vi "New.vi"(1 "Before Write":string) -> (0 "String Writer":refnum<class "String.lvclass">)   [LabVIEW 2018, in "Toolkit.lvlib" / "Writers.lvlib" / "String.lvclass"]
doc: "Creates a new String Writer object.\n\n<B>Before Write</B> - The initial contents of the destination. The rendered Mustache template will be appended to the contents of this value.\n\n<B>String Writer</B> - Represents an implementation capable of writing a rendered Mustache templates to a string."
uses:
  String.lvclass
  String.lvclass/String.ctl
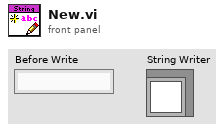
[diagram p1: front panel]
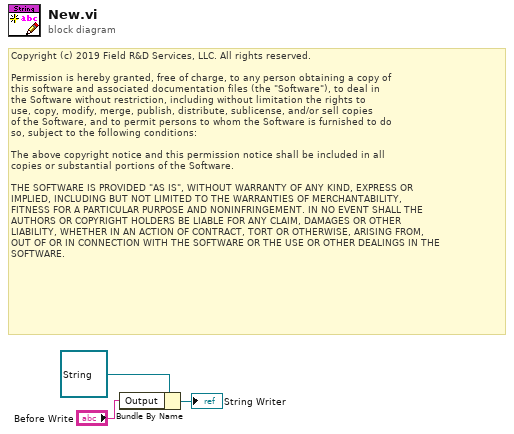
[diagram p0: block diagram]
diagram:
  # "Copyright (c) 2019 Field R&D Services, LLC. All rights reserved.\n\nPermission is hereby granted, free of charge, to any person obtaining a copy of\nthis software and associated documentation files (the \"Software\"), to deal in\nthe Software without restriction, including without limitation the rights to\nuse, copy, modify, merge, publish, distribute, sublicense, and/or sell copies\nof the Software, and to permit persons to whom the Software is furnished to do\nso, subject to the following conditions:\n\nThe above copyright notice and this permission notice shall be included in all\ncopies or substantial portions of the Software.\n\nTHE SOFTWARE IS PROVIDED \"AS IS\", WITHOUT WARRANTY OF ANY KIND, EXPRESS OR\nIMPLIED, INCLUDING BUT NOT LIMITED TO THE WARRANTIES OF MERCHANTABILITY,\nFITNESS FOR A PARTICULAR PURPOSE AND NONINFRINGEMENT. IN NO EVENT SHALL THE\nAUTHORS OR COPYRIGHT HOLDERS BE LIABLE FOR ANY CLAIM, DAMAGES OR OTHER\nLIABILITY, WHETHER IN AN ACTION OF CONTRACT, TORT OR OTHERWISE, ARISING FROM,\nOUT OF OR IN CONNECTION WITH THE SOFTWARE OR THE USE OR OTHER DEALINGS IN THE\nSOFTWARE."
  n1 = Bundle By Name(cluster=refnum<class "String.lvclass"> refnum ("Toolkit.lvlib:Writers.lvlib:String.lvclass"), "Output"="Before Write") -> (→"String Writer":refnum<class "String.lvclass">)
